vi "AMIMonitor_arbeitsversion.vi"   [LabVIEW 2016]
uses:
  Instrument_Setup.vi
  Global/Global Variables/Data_Display_global.vi
types:
  T1 = cluster{"GPIB address":i16, "GPIB bus":i16, "connection ID":refnum<k5>, "IP":string, "Active Comm Interface":u16, "Serial Port":refnum<visa-resource-name>, "Programmer Type":u16}
  T2 = cluster{"error":bool, "code":i32, "source":string}
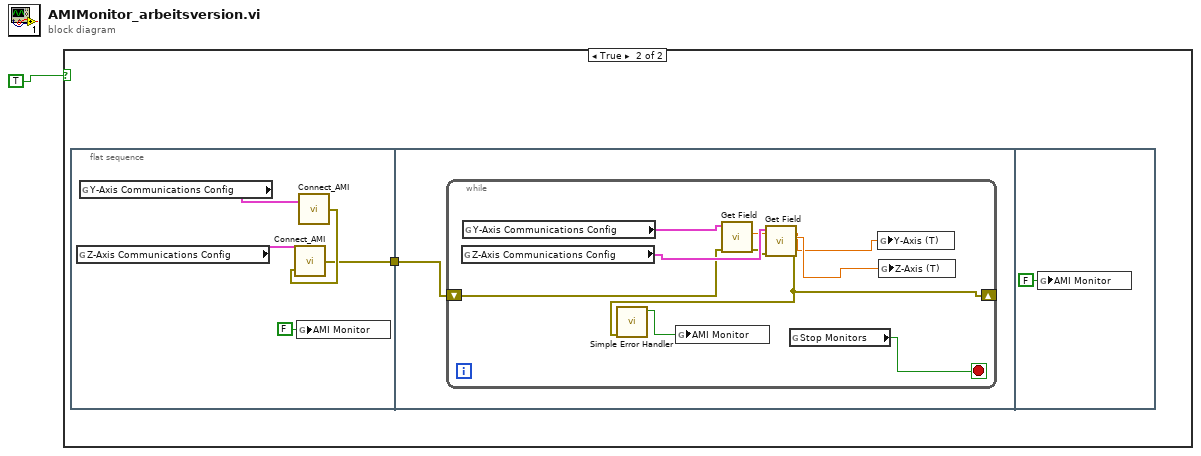
[diagram p0: block diagram]
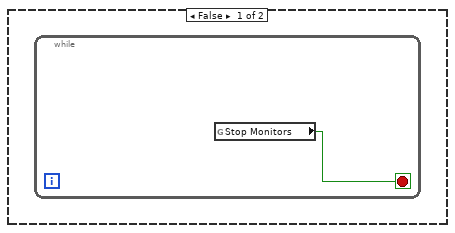
[diagram p2: hidden frame]
diagram:
  n1 = case shown="True" TRUE {
    frame False {
      n2 = while {
        stop <- w2 stop-if-true
        n3 = global read "Data_Display_global.vi" "Stop Monitors"() -> (w2:bool)
      }
    }
    frame True {
      n4 = flat-sequence {
        tunnel: [w4] -> w3
        tunnel: w3 -> [w9]
        frame #0 {
          n5 = global read "Instrument_Setup.vi" "Z-Axis Communications Config"() -> (w6:T1)
          n6 = global read "Instrument_Setup.vi" "Y-Axis Communications Config"() -> (w7:T1)
          n7 = global write "Data_Display_global.vi" "AMI Monitor"(FALSE) -> ()
          n8 = call "Connect_AMI.vi"("Communications Config"=w7) -> ("error out"=w5:T2)  [unwired: 1 in]
          n9 = call "Connect_AMI.vi"("error in"=w5, "Communications Config"=w6) -> ("error out"=w4:T2)
        }
        frame #1 {
          n10 = while {
            shift-right: [w10] -> _
            shift-left: w9 -> [w11]
            stop <- w18 stop-if-true
            n11 = global read "Instrument_Setup.vi" "Z-Axis Communications Config"() -> (w15:T1)
            n12 = global read "Instrument_Setup.vi" "Y-Axis Communications Config"() -> (w16:T1)
            n13 = call "Get Field.vi"("Z-Axis Communications Config"=w16, "error in"=w11) -> ("Field(T)"=w13:dbl, "error out"=w12:T2)  [unwired: 4 in, 1 out]
            n14 = call "Get Field.vi"("Z-Axis Communications Config"=w15, "error in"=w12) -> ("Field(T)"=w14:dbl, "error out"=w10:T2)  [unwired: 4 in, 1 out]
            n15 = call <vilib>:"Simple Error Handler.vi"("error in (no error)"=w10) -> ("error?"=w17:bool)  [unwired: 4 in, 4 out]
            n16 = global write "Data_Display_global.vi" "AMI Monitor"(w17) -> ()
            n17 = global read "Data_Display_global.vi" "Stop Monitors"() -> (w18:bool)
            n18 = global write "Data_Display_global.vi" "Y-Axis (T)"(w13) -> ()
            n19 = global write "Data_Display_global.vi" "Z-Axis (T)"(w14) -> ()
          }
        }
        frame #2 {
          n20 = global write "Data_Display_global.vi" "AMI Monitor"(FALSE) -> ()
        }
      }
    }
  }
